vi "DotProduct.vi"(8 "error in (no error)":errorcluster, 9 "Point2":dbl[](array[numeric]), 10 "Point1":dbl[](array[numeric]), 11 "object in":refnum<class "Utilities.lvclass">) -> (0 "error out":errorcluster, 2 "dot product":dbl, 3 "object out":refnum<class "Utilities.lvclass">)   [LabVIEW 2023, in "Utilities.lvclass"]
uses:
  Utilities.lvclass
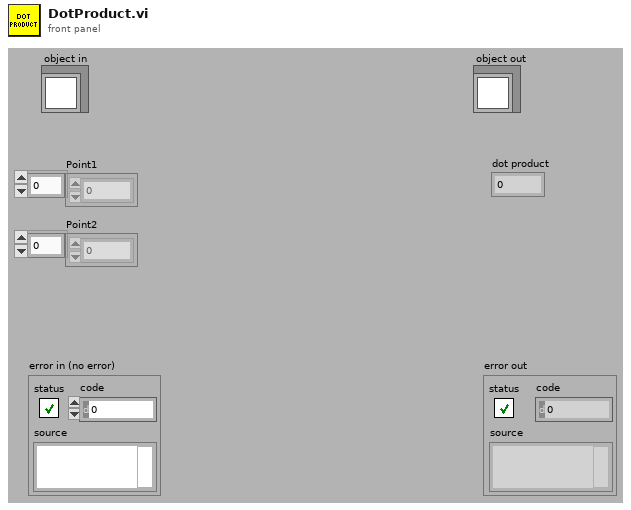
[diagram p1: front panel]
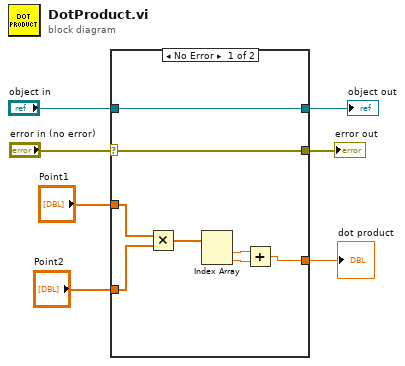
[diagram p0: block diagram]
diagram:
  n1 = case shown="No Error" "error in (no error)" {
    selector: "error in (no error)" -> [w15 w17]
    tunnel: [w15 w17] -> w6
    tunnel: [w14 w16] -> w4
    tunnel: "object in" -> [w14 w16]
    tunnel: "Point1" -> [w13 _]
    tunnel: "Point2" -> [w12 _]
    tunnel: [w8 _] -> w1
    frame No Error {
      n2 = Multiply(x=w13, y=w12) -> (x*y=w11:dbl[])
      n3 = Index Array(array=w11) -> (element #1=w10:dbl, element #2=w9:dbl)  [unwired: 2 in]
      n4 = Add(x=w10, y=w9) -> (x+y=w8:dbl)
    }
    frame Error {
    }
  }
  "error out" <- w6
  "object out" <- w4
  "dot product" <- w1
